vi "Write clock rate.vi"(8 "error in (no error)":errorcluster, 10 "clock rate":dbl=1200000000.0, 11 "build_waveform in":refnum<class "build_waveform.lvclass">) -> (0 "error out":errorcluster, 3 "build_waveform out":refnum<class "build_waveform.lvclass">)   [LabVIEW 2015, in "build_waveform.lvclass"]
uses:
  build_waveform.lvclass
  build_waveform.lvclass/build_waveform.ctl
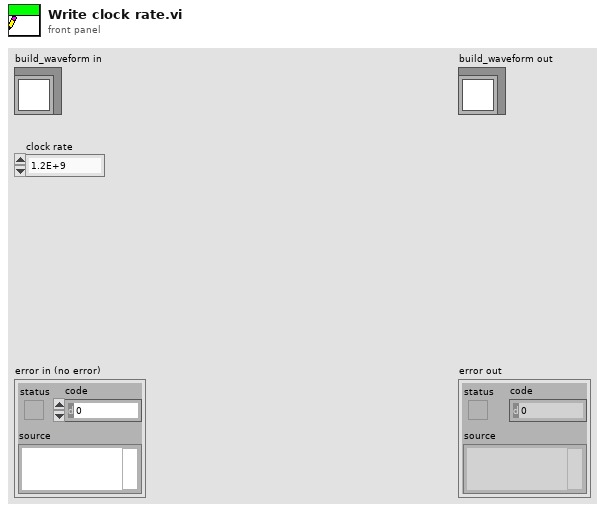
[diagram p1: front panel]
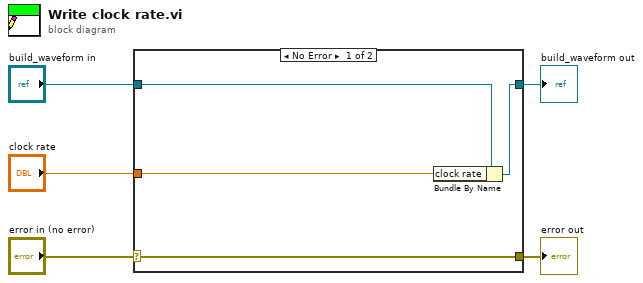
[diagram p0: block diagram]
diagram:
  n1 = case shown="No Error" "error in (no error)" {
    selector: "error in (no error)" -> [w9 w10]
    tunnel: [w9 w10] -> w4
    tunnel: [w7 w11] -> w2
    tunnel: "build_waveform in" -> [w8 w11]
    tunnel: "clock rate" -> [w6 _]
    frame No Error {
      n2 = Bundle By Name(cluster=w8, "clock rate"=w6) -> (w7:refnum<class "build_waveform.lvclass">)
    }
    frame Error {
    }
  }
  "error out" <- w4
  "build_waveform out" <- w2
